vi "ALTS-2015 Force Scan.vi"(8 "error in (no error)":errorcluster, 10 "Timeout?":bool, 11 "FIFO_Task Details":T1) -> (0 "error out":errorcluster, 3 "Task Details_Out":T1)   [LabVIEW 2013]
uses:
  Controls/ALTS-2015 Serial Details.ctl
  Controls/ALTS-2015 Robot Tasks.ctl
  Controls/ALTS-2015 Station Cluster.ctl
  Controls/ALTS-2015 Serial DB Details.ctl
  Controls/ALTS-2015 Status Message Options.ctl
  Controls/ALTS-2015 DB Driver Options.ctl
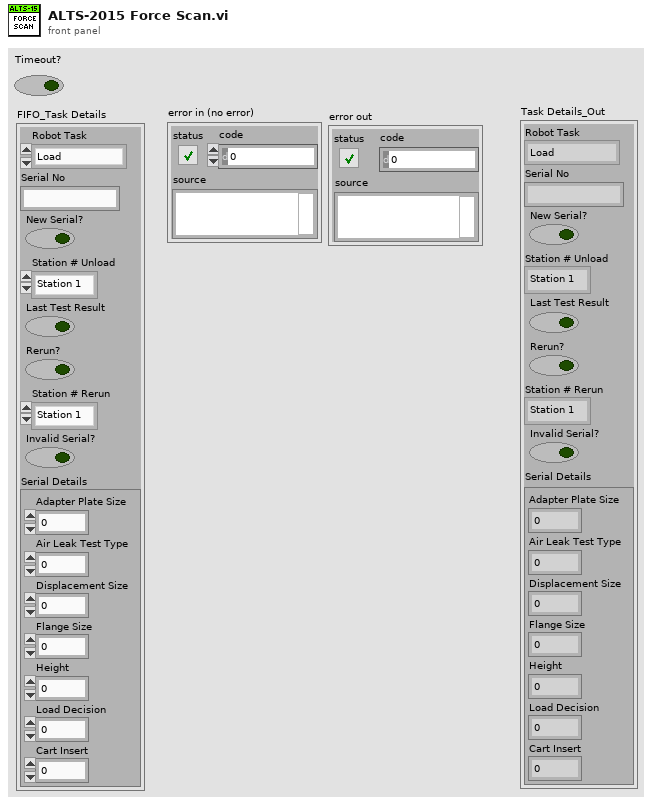
[diagram p1: front panel]
types:
  T1 = typedef "ALTS-2015 Serial Details.ctl" = cluster{"Robot Task":T2, "Serial No":string, "New Serial?":bool, "Station # Unload":T3, "Last Test Result":bool, "Rerun?":bool, "Station # Rerun":T3, "Invalid Serial?":bool, "Serial Details":T4}
  T2 = typedef "ALTS-2015 Robot Tasks.ctl" = enum16{"Load", "Unload", "Rerun", "Invalid Serial"}
  T3 = typedef "ALTS-2015 Station Cluster.ctl" = enum16{"Station 1", "Station 2", "Station 3", "Station 4"}
  T4 = typedef "ALTS-2015 Serial DB Details.ctl" = cluster{"Adapter Plate Size":i32, "Air Leak Test Type ":i32, "Displacement Size":i32, "Flange Size":i32, "Height":i32, "Load Decision":i32, "Cart Insert":i32}
  T5 = typedef "ALTS-2015 Status Message Options.ctl" = enum16{"Initializing...", "Enter User Login...", "Valid Serial Number...", "Invalid Serial Number...", "Start Tag Received...", "Stop Tag Received...", "UUT Clamped...", "UUT not Clamped...", "Test Running...", "Test Complete...", "Task is assigned to robot...", "Robot is working on the task...", "Robot is ready for next task...", "Writing Result to DB...", "Idle...", "Exiting..."}
  T6 = typedef "ALTS-2015 DB Driver Options.ctl" = enum16{"Init", "Read DB", "Close"}
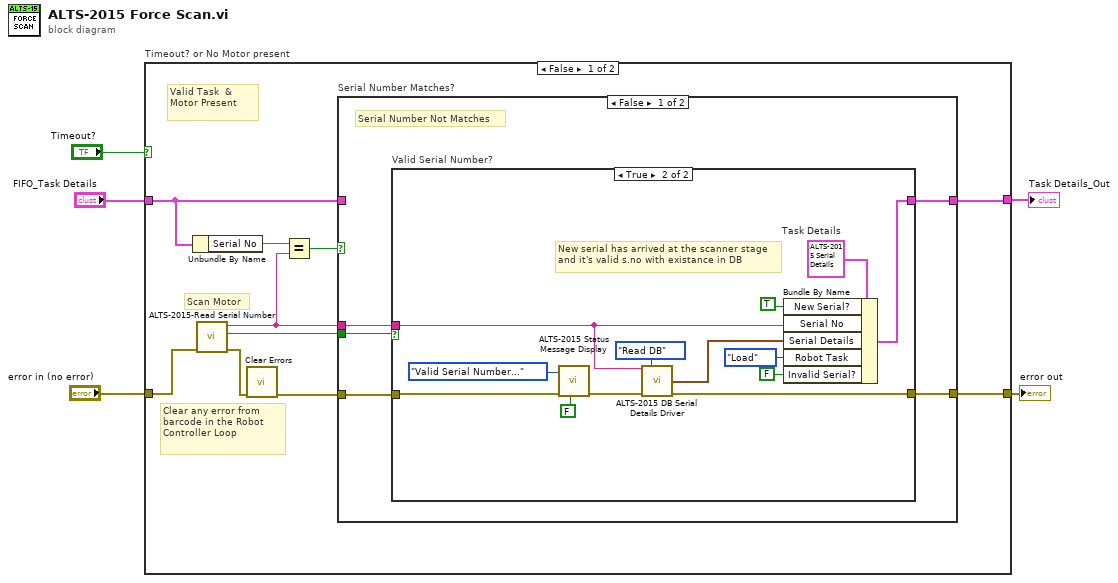
[diagram p0: block diagram]
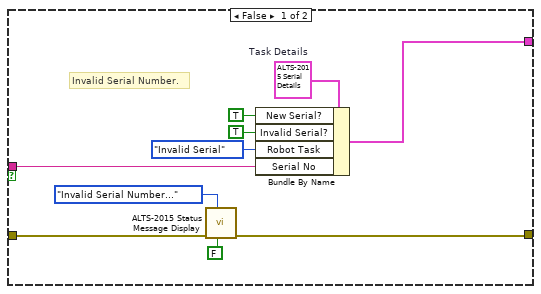
[diagram p2: hidden frame]
diagram:
  n1 = case "Timeout? or No Motor present" shown="False" "Timeout?" {
    tunnel: [w12 w46] -> w5
    tunnel: [w11 w47] -> w2
    tunnel: "FIFO_Task Details" -> [w7 w47]
    tunnel: "error in (no error)" -> [w6 w46]
    frame False {
      # "Valid Task  & Motor Present"
      # "Scan Motor"
      # "Clear any error from barcode in the Robot Controller Loop"
      n2 = Unbundle By Name(w7) -> ("Serial No"=w10:string)
      n3 = call "ALTS-2015-Read Serial Number.vi"("error in (no error)"=w6) -> ("error out"=w14:errorcluster, "Valid Serial Number?"=w15:bool, "Serial No"=w9:string)  [unwired: 8 in]
      n4 = call <vilib>:"Clear Errors.vi"("error in (no error)"=w14) -> ("error out"=w13:errorcluster)  [unwired: 6 in]
      n5 = Equal?(x=w10, y=w9) -> (x = y?=w8:bool)
      n6 = case "Serial Number Matches?" shown="False" w8 {
        tunnel: w15 -> [w20 _]
        tunnel: w13 -> [w19 w44]
        tunnel: [w18 w44] -> w12
        tunnel: [w17 w45] -> w11
        tunnel: w9 -> [w16 _]
        tunnel: w7 -> [_ w45]
        frame False {
          # "Serial Number Not Matches"
          n7 = case "Valid Serial Number?" shown="True" w20 {
            tunnel: w19 -> [w29 w41]
            tunnel: w16 -> [w22 w33]
            tunnel: [w27 w32] -> w18
            tunnel: [w21 w31] -> w17
            frame False {
              w26 = T1 {"Robot Task"=enum."Load", "Serial No"="", "New Serial?"=FALSE, "Station # Unload"=enum."Station 1", "Last Test Result"=FALSE, "Rerun?"=FALSE, "Station # Rerun"=enum."Station 1", "Invalid Serial?"=FALSE, "Serial Details"={"Adapter Plate Size"=0, "Air Leak Test Type "=0, "Displacement Size"=0, "Flange Size"=0, "Height"=0, "Load Decision"=0, "Cart Insert"=0}}  # Task Details
              # "Invalid Serial Number."
              n8 = call "ALTS-2015 Status Message Display.vi"("Station Message?"=FALSE, "Status Message Options"=ALTS-2015_Status_Message_Options."Invalid Serial Number...", "error in (no error)"=w29) -> ("error out"=w27:errorcluster)  [unwired: 7 in, 1 out]
              n9 = Bundle By Name(cluster=w26, "New Serial?"=TRUE ("New Part?"), "Invalid Serial?"=TRUE, "Robot Task"=ALTS-2015_Robot_Tasks."Invalid Serial", "Serial No"=w22) -> (w21:T1)
            }
            frame True {
              w37 = T1 {"Robot Task"=enum."Load", "Serial No"="", "New Serial?"=FALSE, "Station # Unload"=enum."Station 1", "Last Test Result"=FALSE, "Rerun?"=FALSE, "Station # Rerun"=enum."Station 1", "Invalid Serial?"=FALSE, "Serial Details"={"Adapter Plate Size"=0, "Air Leak Test Type "=0, "Displacement Size"=0, "Flange Size"=0, "Height"=0, "Load Decision"=0, "Cart Insert"=0}}  # Task Details
              # "New serial has arrived at the scanner stage\nand it's valid s.no with existance in DB"
              n10 = call "ALTS-2015 Status Message Display.vi"("Station Message?"=FALSE, "Status Message Options"=ALTS-2015_Status_Message_Options."Valid Serial Number...", "error in (no error)"=w41) -> ("error out"=w34:errorcluster)  [unwired: 7 in, 1 out]
              n11 = call "ALTS-2015 DB Serial Details Driver.vi"("Serial Number"=w33, "Operation"=ALTS-2015_DB_Driver_Options."Read DB", "error in (no error)"=w34) -> ("Serial Details from DB"=w36:T4, "error out"=w32:errorcluster)  [unwired: 10 in, 1 out]
              n12 = Bundle By Name(cluster=w37, "New Serial?"=TRUE ("New Part?"), "Serial No"=w33, "Serial Details"=w36, "Robot Task"=ALTS-2015_Robot_Tasks."Load", "Invalid Serial?"=FALSE) -> (w31:T1)
            }
          }
        }
        frame True {
          # "Serial Number Matches"
        }
      }
    }
    frame True {
    }
  }
  "error out" <- w5
  "Task Details_Out" <- w2
